vi "run.update.path.vi"(8 "error in":errorcluster, 10 "rid":string) -> (0 "error out":errorcluster, 3 "path":string)   [LabVIEW 2020, in "Nominal Client.lvclass"]
uses:
  Nominal Client.lvclass
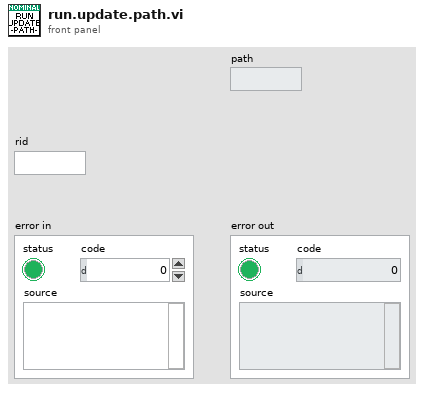
[diagram p1: front panel]
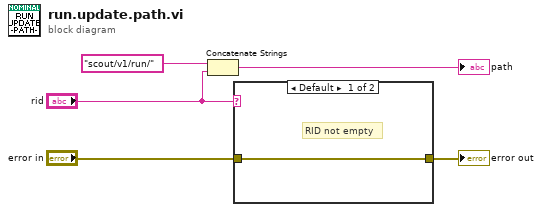
[diagram p0: block diagram]
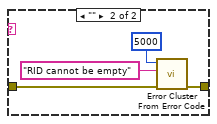
[diagram p2: hidden frame]
diagram:
  n1 = Concatenate Strings("scout/v1/run/" ("Path"), "rid") -> (→"path":string)
  n2 = case shown="Default" "rid" {
    tunnel: "error in" -> [w6 w9]
    tunnel: [w6 w8] -> w1
    frame Default {
      # "RID not empty"
    }
    frame "" {
      n3 = call <vilib>:"Error Cluster From Error Code.vi"("error in (no error)"=w9, "error message (\"\")"="RID cannot be empty" ("error message (\"\")"), "error code (0)"=5000) -> ("error out"=w8:errorcluster)  [unwired: 6 in]
    }
  }
  "error out" <- w1
